vi "AF_4.0.0_Actor Core1.vi"(8 "error in":errorcluster, 11 "Actor in":refnum<class "Actor1_GUI_N_4.0.0.lvclass">) -> (0 "error out":errorcluster, 3 "Actor out(KEEP)":refnum<class "Actor.lvclass">)   [LabVIEW 2020]
doc: "This is Actor Core.vi, the main message handling loop for Actors. An actor usually just sits in this loop and processes messages as they arrive. Any error returned by the message Do.vi call will stop the loop, with error code 43 as the cannonical signal to stop with no error sent to caller. Descendants may override that in Handle Error.vi."
uses:
  <vilib>/ActorFramework/Actor/Actor.lvclass
  <resource>/Framework/Providers/Open_GDS/ClassProviders/ActorFramework/4.0.0/Actor1_GUI_N_4.0.0/Actor1_GUI_N_4.0.0_class/Actor1_GUI_N_4.0.0.lvclass
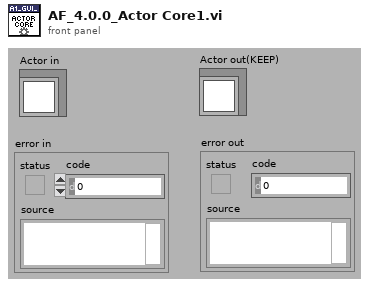
[diagram p1: front panel]
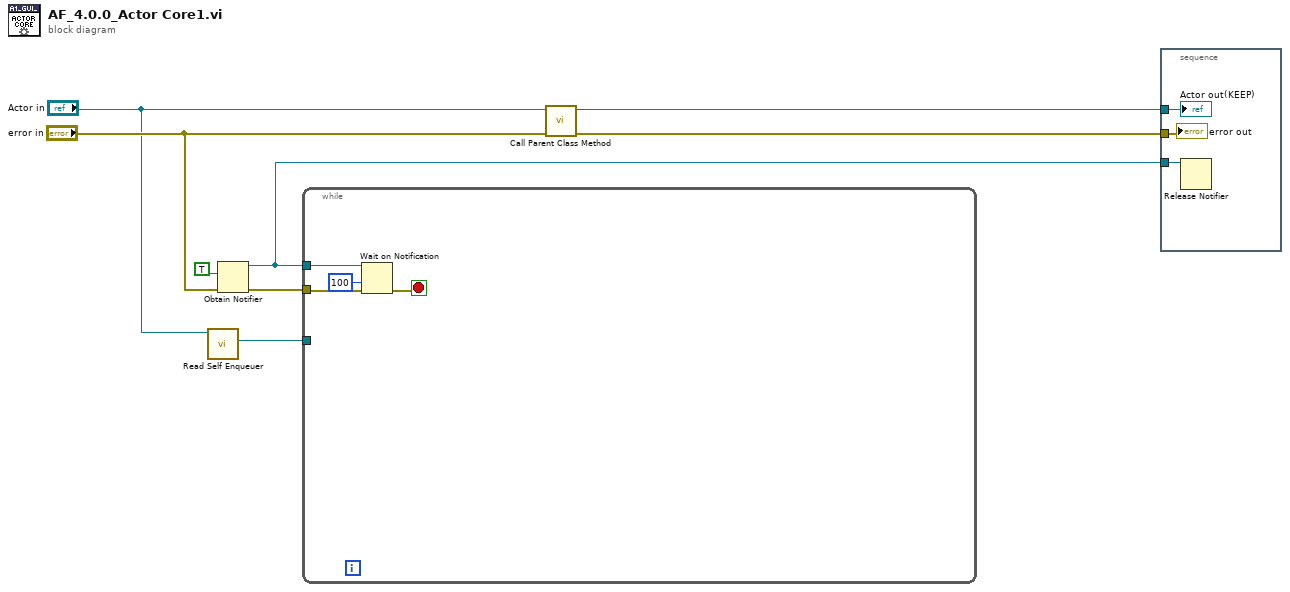
[diagram p0: block diagram]
diagram:
  n1 = call <vilib>:"Read Self Enqueuer.vi"("Actor"="Actor in") -> ("Self Enqueuer"=w2:refnum<class "Message Enqueuer.lvclass">)  [unwired: 10 in]
  n2 = Obtain Notifier(notification data type=TRUE, error in (no error)="error in") -> (notifier out=w3:refnum<notifier>, error out=w6:errorcluster)  [unwired: 2 in, 1 out]
  n3 = while {
    tunnel: w6 -> [w12]
    tunnel: w3 -> [w11]
    tunnel: w2 -> [_]
    stop <- w10 stop-if-true
    n4 = Wait on Notification(notifier=w11, timeout in ms (-1)=100, error in (no error)=w12) -> (error out=w10:errorcluster)  [unwired: 1 in, 3 out]
  }
  n5 = call-parent "Call Parent Class Method"("error in"="error in", "Actor"="Actor in") -> ("error out"=w4:errorcluster, "Actor out"=w8:refnum<class "Actor.lvclass">)  [unwired: 8 in]
  n6 = stacked-sequence {
    tunnel: w8 -> [w15]
    tunnel: w4 -> [w14]
    tunnel: w3 -> [w13]
    frame #0 {
      n7 = Release Notifier(notifier=w13) -> ()  [unwired: 2 in, 3 out]
      "Actor out(KEEP)" <- w15
      "error out" <- w14
    }
  }
